vi "Inv Chebyshev Coefficients.vi"(5 "filter structure option":T1=10 items=["IIR 2nd Order"=0, "IIR 4th Order"=1, "Auto Select"=10], 6 "order":i32=2, 7 "filter type":T3, 8 "attenuation (dB)":dbl=60.0 format="%0.2f", 9 "low cutoff freq: fl":dbl=0.125 format="%0.3f", 10 "high cutoff freq: fh":dbl=0.45000000000000007 format="%0.2f", 11 "sampling freq: fs":dbl=1.0 format="%0.2f") -> (0 "error":i32, 3 "IIR Filter Cluster":T2 {"Forward Coefficients" format="%.4f"; "Reverse Coefficients" format="%.4f"})   [LabVIEW 2010, in "NI_AALBase.lvlib"]
doc: "Generates the set of filter coefficients to implement an IIR filter as specified by the Chebyshev II Filter model."
uses:
  NI_AALBase.lvlib
  Filter Passband Type.ctl
  Filter Structure Type.ctl
  lvanlys.dll
panel:
  # "Inverse Chebyshev Coefficients"
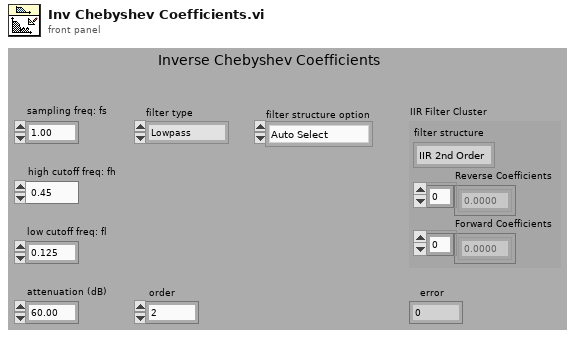
[diagram p1: front panel]
types:
  T1 = typedef "NI_AALBase.lvlib/Filter Structure Type.ctl" = u16
  T2 = cluster{"filter structure":enum32{"IIR 2nd Order", "IIR 4th Order"}, "Reverse Coefficients":dbl[], "Forward Coefficients":dbl[]}
  T3 = typedef "NI_AALBase.lvlib/Filter Passband Type.ctl" = enum32{"Lowpass", "Highpass", "Bandpass", "Bandstop"}
  T4 = cluster{"filter structure":enum32{"IIR 2nd Order", "IIR 4th Order"}, "aH":dbl[], "bH":dbl[]}
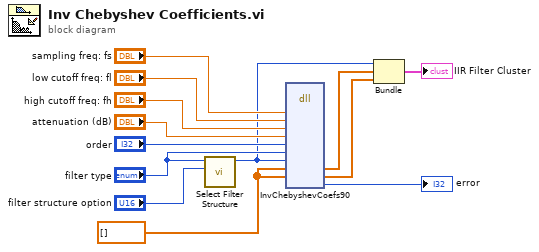
[diagram p0: block diagram]
diagram:
  w8 = dbl[] [] ("[DBL]")
  n1 = call "Select Filter Structure.vi"("filter structure option"="filter structure option", "filter type"="filter type") -> ("filter structure"=w1:enum32{"IIR 2nd Order", "IIR 4th Order"})  [unwired: 9 out]
  n2 = dll-call lib="C:/Program Files/National Instruments/LabVIEW 2010/resource/lvanlys.*" fn="InvChebyshevCoefs90"("fs"="sampling freq: fs", "fl"="low cutoff freq: fl", "fh"="high cutoff freq: fh", "r"="attenuation (dB)", "order"="order", "type"="filter type", "structure"=w1, "aH"=w8, "bH"=w8) -> ("aH"=w6:dbl[], "bH"=w5:dbl[], "dsperr"=→"error":i32)  [unwired: 9 in, 5 out]
  n3 = Bundle("filter structure"=w1, "aH"=w6, "bH"=w5) -> (→"IIR Filter Cluster":T4)  [unwired: 1 out]
